vi "TestLimelight.vi"() -> ()   [LabVIEW 2018]
uses:
  Limelight.llb/LL_LEDSetValue.ctl
  Limelight.llb/LL_TargetData.ctl
  Limelight.llb/Limelight.lvclass/Limelight.ctl
  Limelight.llb/Limelight.lvclass
panel:
  out "Target Data":T1
  in  "stop":bool
  in  "LEDSetValue":T2=enum."Override Off"
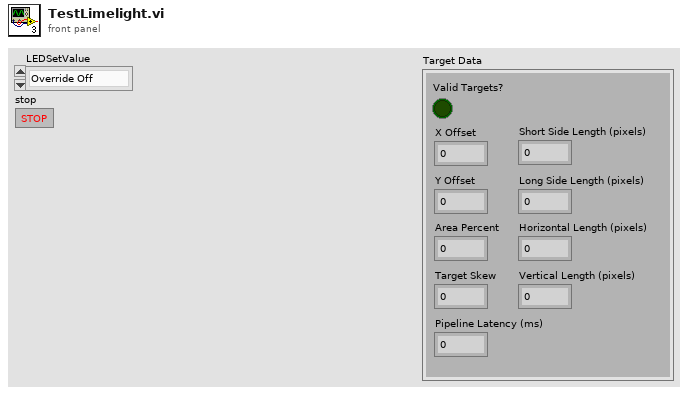
[diagram p1: front panel]
types:
  T1 = typedef "Limelight.lvclass/LL_TargetData.ctl" = cluster{"Valid Targets?":bool, "X Offset":dbl, "Y Offset":dbl, "Area Percent":dbl, "Target Skew":dbl, "Short Side Length (pixels)":dbl, "Long Side Length (pixels)":dbl, "Horizontal Length (pixels)":dbl, "Vertical Length (pixels)":dbl, "Pipeline Latency (ms)":dbl}
  T2 = typedef "Limelight.lvclass/LL_LEDSetValue.ctl" = enum16{"Pipeline Default", "Override Off", "Override Blink", "Override On"}
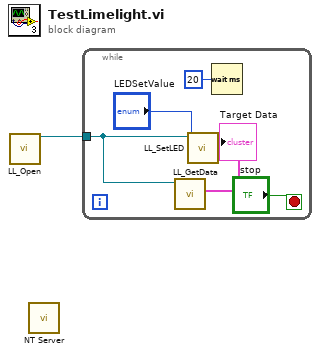
[diagram p0: block diagram]
diagram:
  n1 = call "LL_Open.vi"() -> ("Limelight out"=w1:refnum<class "Limelight.lvclass">)  [unwired: 10 in, 1 out]
  n2 = call <vilib>:"NT Server.vi"() -> ()  [unwired: 12 in]
  n3 = while {
    tunnel: w1 -> [w4]
    stop <- "stop" stop-if-true
    n4 = call "LL_GetData.vi"("Limelight in"=w4) -> ("Target Data"=→"Target Data":T1)  [unwired: 8 in, 2 out]
    n5 = call "LL_SetLED.vi"("LEDSetValue"="LEDSetValue", "Limelight in"=w4) -> ()  [unwired: 8 in, 2 out]
    n6 = Wait (ms)(milliseconds to wait=u32 20) -> ()  [unwired: 1 out]
  }
